vi "Read ID.vi"(8 "error in (no error)":errorcluster, 11 "ConnectionManager in":refnum<class "ConnectionManager.lvclass">) -> (0 "error out":errorcluster, 2 "ID":string, 3 "ConnectionManager out":refnum<class "ConnectionManager.lvclass">)   [LabVIEW 2020, in "ConnectionManager.lvlib" / "ConnectionManager.lvclass"]
uses:
  <vilib>/gpm_packages/@cs/Network-interface/Source/ConnectionManager/ConnectionManager/ConnectionManager.lvclass
  <vilib>/gpm_packages/@cs/Network-interface/Source/ConnectionManager/ConnectionManager/ConnectionManager.lvclass/ConnectionManager.ctl
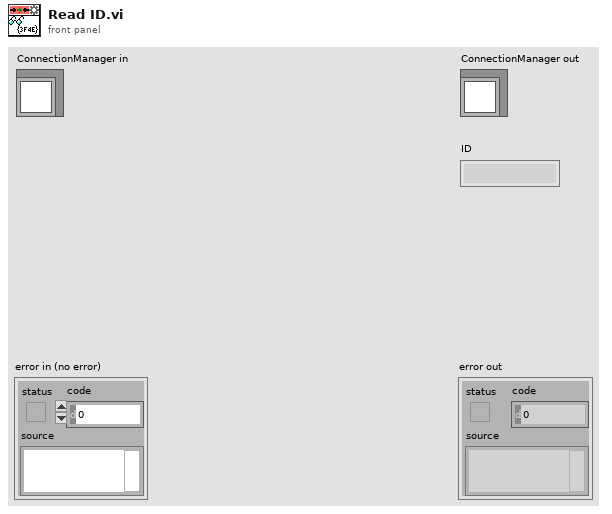
[diagram p1: front panel]
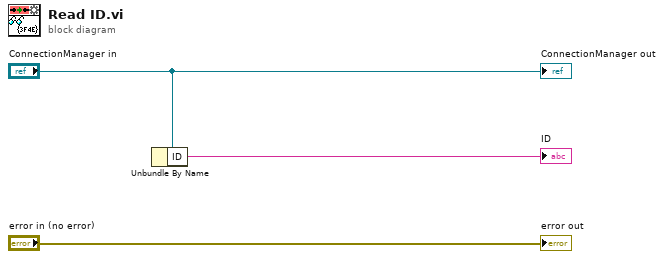
[diagram p0: block diagram]
diagram:
  n1 = Unbundle By Name("ConnectionManager in") -> ("ID"=→"ID":string)
  "error out" <- "error in (no error)"
  "ConnectionManager out" <- "ConnectionManager in"
